vi "CRYDataView Pos In Bound.vi"(8 "Mouse Pos":T1, 11 "Ref In":refnum<vi>) -> (3 "bResult":bool)   [LabVIEW 2013]
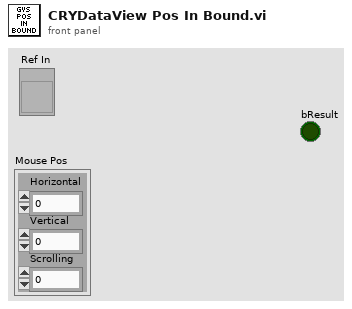
[diagram p1: front panel]
types:
  T1 = cluster{"Horizontal":i32, "Vertical":i32, "Scrolling":i32}
  T2 = typedef "LVRectTypeDef.ctl" = cluster{"Left":i16, "Top":i16, "Right":i16, "Bottom":i16}
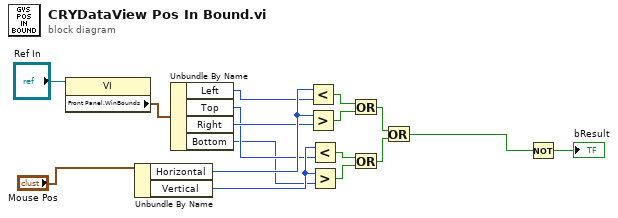
[diagram p0: block diagram]
diagram:
  n1 = property class="VI"(reference="Ref In") -> ("Front Panel.WinBounds"=w9:T2)  [unwired: 1 in, 2 out]
  n2 = Unbundle By Name("Mouse Pos") -> ("Horizontal"=w16:i32, "Vertical"=w17:i32)
  n3 = Unbundle By Name(w9) -> ("Left"=w8:i16, "Top"=w6:i16, "Right"=w7:i16, "Bottom"=w5:i16)
  n4 = Less?(x=w16, y=w8) -> (x < y?=w11:bool)
  n5 = Greater?(x=w16, y=w7) -> (0:w15:bool)
  n6 = Less?(x=w17, y=w6) -> (x < y?=w14:bool)
  n7 = Greater?(x=w17, y=w5) -> (0:w10:bool)
  n8 = Or(x=w11, y=w15) -> (x .or. y?=w12:bool)
  n9 = Or(x=w14, y=w10) -> (x .or. y?=w13:bool)
  n10 = Or(x=w12, y=w13) -> (x .or. y?=w4:bool)
  n11 = Not(x=w4) -> (.not. x?=→"bResult":bool)
